vi "Write Multiple to String Log.vi"(10 "Strings to Log":string[](array[string]), 11 "String Log Sink in":refnum<class "String Log Sink.lvclass">) -> (0 "error out":errorcluster, 3 "String Log Sink out":refnum<class "String Log Sink.lvclass">)   [LabVIEW 2019, in "String Log Sink.lvclass"]
uses:
  String Log Sink.lvclass
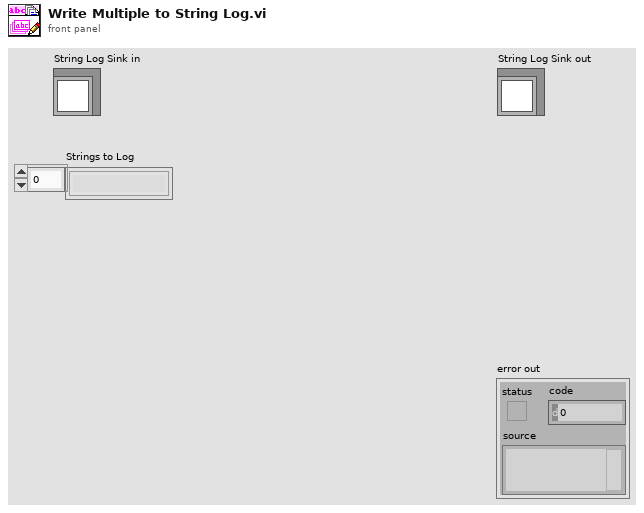
[diagram p1: front panel]
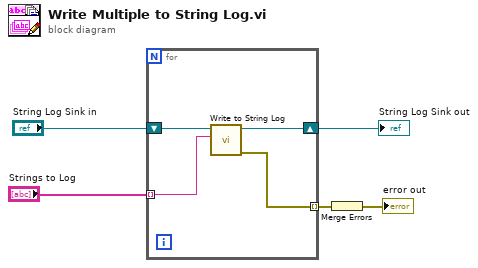
[diagram p0: block diagram]
diagram:
  n1 = for {
    shift-right: [w8] -> w4
    shift-left: "String Log Sink in" -> [w9]
    tunnel: "Strings to Log" -> [w7] mode=indexing
    tunnel: [w6] -> w1 mode=indexing
    n2 = call-dynamic "Write to String Log.vi"("String to Log"=w7, "String Log Sink in"=w9) -> ("error out"=w6:errorcluster, "String Log Sink out"=w8:refnum<class "String Log Sink.lvclass">)  [unwired: 8 in]
  }
  "String Log Sink out" <- w4
  n3 = Merge Errors(w1) -> (→"error out":errorcluster)
